vi "Default MQTT Packet (Empty).vi"() -> (3 "No Packet":refnum<class "ControlPacket.lvclass">)   [LabVIEW 2013]
uses:
  ControlPacket.lvclass
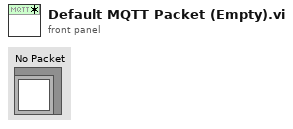
[diagram p1: front panel]
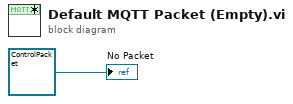
[diagram p0: block diagram]
diagram:
  "No Packet" <- refnum<class "ControlPacket.lvclass"> refnum ("t")
